vi "Test API No Error Running Tests in Empty Library.vi"(8 "error in (no error)":errorcluster, 11 "API Test in":refnum<class "API Test.lvclass">) -> (0 "error out":errorcluster, 3 "API Test out":refnum<class "API Test.lvclass">)   [LabVIEW 2020, in "LUnit Tests.lvlib" / "API Test.lvclass"]
uses:
  API Test.lvclass
  source/Framework/Execution API/Execution API.lvclass
  <vilib>/Astemes/LUnit/Test Case.lvclass
  C:/Program Files (x86)/National Instruments/LabVIEW 2021/vi.lib/Astemes/LUnit/Test Case.lvclass
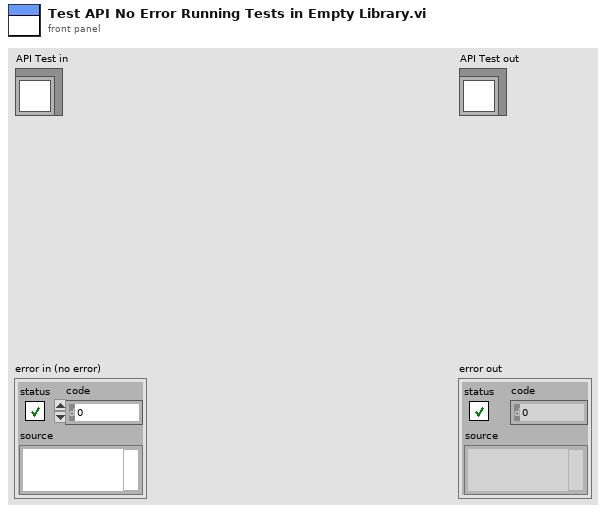
[diagram p1: front panel]
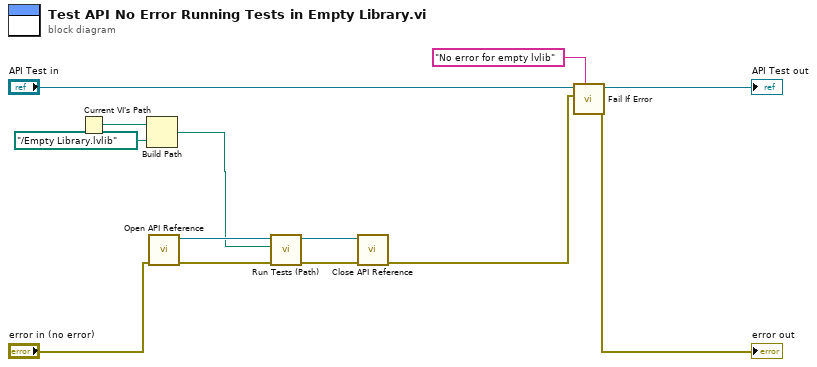
[diagram p0: block diagram]
diagram:
  n1 = Current VI's Path() -> (path=w3:path)
  n2 = Build Path(base path=w3, name or relative path=path "../Empty Library.lvlib") -> (appended path=w1:path)
  n3 = call "Open API Reference.vi"("error in (no error)"="error in (no error)") -> ("error out"=w12:errorcluster, "Execution API out"=w13:refnum<class "Execution API.lvclass">)  [unwired: 9 in]
  n4 = call "Run Tests (Path).vi"("error in (no error)"=w12, "Project or Class Path"=w1, "Execution API In"=w13) -> ("error out"=w11:errorcluster, "Execution API Out"=w10:refnum<class "Execution API.lvclass">)  [unwired: 7 in]
  n5 = call "Close API Reference.vi"("error in (no error)"=w11, "Execution API in"=w10) -> ("error out"=w6:errorcluster)  [unwired: 9 in]
  n6 = call <vilib>:"Fail If Error.vi"("Description"="No error for empty lvlib", "Assert error"=w6, "LUnit Test Case In"="API Test in") -> ("error out"=→"error out":errorcluster, "LUnit Test Case Out"=→"API Test out":refnum<class "API Test.lvclass">)  [unwired: 7 in]
